vi "grep.vi"(10 "Keyword (Regular Expression)":string="TOTEN  =", 11 "File String":string) -> (3 "Result":string[](array[string]))   [LabVIEW 2010]
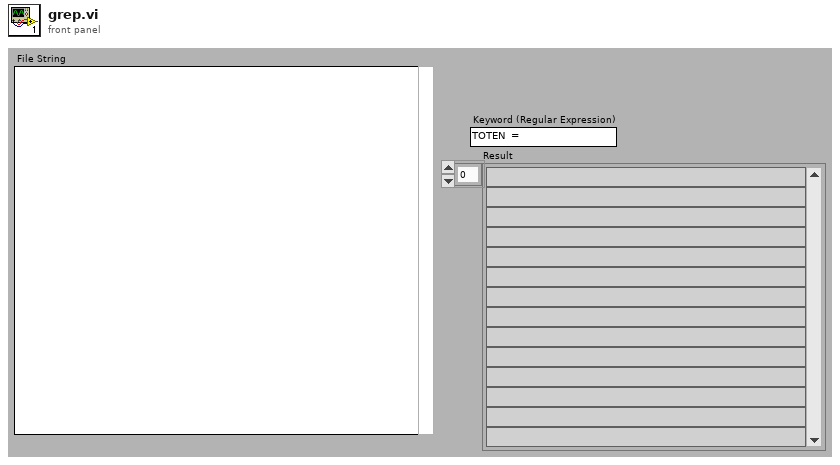
[diagram p1: front panel]
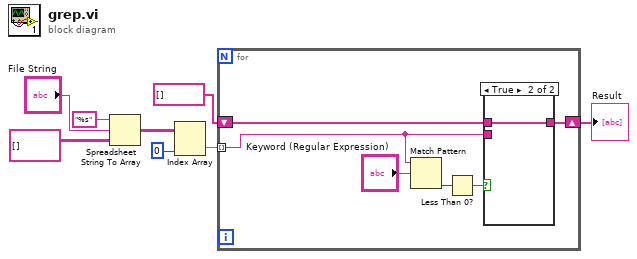
[diagram p0: block diagram]
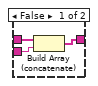
[diagram p2: hidden frame]
diagram:
  n1 = Spreadsheet String To Array(format string="%s", spreadsheet string="File String", array type (2D Dbl)=string[][] []) -> (array=w3:string[][])  [unwired: 1 in]
  n2 = Index Array(array=w3, index (col)=0 ("disabled index (col)")) -> (element=w1:string[])  [unwired: 1 in]
  n3 = for {
    tunnel: w1 -> [w12] mode=indexing
    shift-right: [w11] -> w4
    shift-left: string[] [] -> [w10]
    n4 = Match Pattern(string=w12, regular expression="Keyword (Regular Expression)") -> (offset past match=w13:i32)  [unwired: 1 in, 3 out]
    n5 = Less Than 0?(x=w13) -> (x < 0?=w9:bool)
    n6 = case shown="True" w9 {
      tunnel: w12 -> [w17 _]
      tunnel: [w16 w18] -> w11
      tunnel: w10 -> [w15 w18]
      frame False {
        n7 = Build Array (concatenate)(w15, w17) -> (w16:string[])
      }
      frame True {
      }
    }
  }
  "Result" <- w4
